vi "Read.vi"(8 "error in":errorcluster, 11 "VISA resource name":refnum<visa-resource-name>) -> (0 "error out":errorcluster, 2 "Message":string, 3 "VISA resource name out":refnum<visa-resource-name>)   [LabVIEW 2019, in "Andeen-Hagerling 2700(400 firmware).lvlib"]
doc: "Read all available bytes from the selected VISA resource."
uses:
  Andeen-Hagerling 2700(400 firmware).lvlib
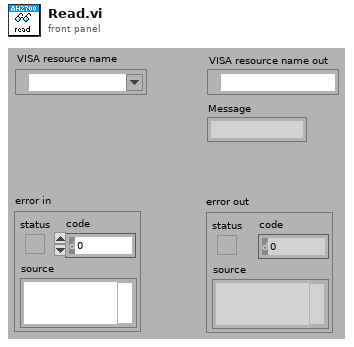
[diagram p1: front panel]
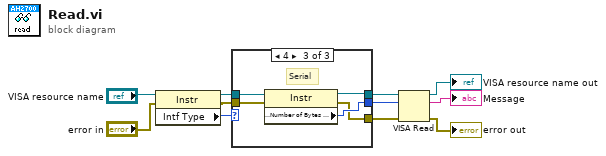
[diagram p0: block diagram]
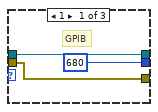
[diagram p2: hidden frame]
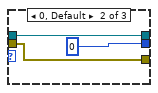
[diagram p3: hidden frame]
diagram:
  n1 = property class="Instr"(reference="VISA resource name", error in="error in") -> (reference out=w10:refnum<visa-resource-name>, error out=w4:errorcluster, "Intf Type"=w11:u16)
  n2 = case shown="4" w11 {
    tunnel: w10 -> [w13 w17 w22]
    tunnel: [w13 w17 w20] -> w9
    tunnel: [w12 w15 w19] -> w8
    tunnel: [u16 680 ("y") u32 0 ("Bytes at Port") w21] -> w7
    tunnel: w4 -> [w12 w15 w18]
    frame 1 {
      # "GPIB"
    }
    frame 0, Default {
    }
    frame 4 {
      # "Serial"
      n3 = property class="Instr"(reference=w22, error in=w18) -> (reference out=w20:refnum<visa-resource-name>, error out=w19:errorcluster, "Serial Settings:Number of Bytes at Serial Port"=w21:u32)
    }
  }
  n4 = VISA Read(VISA resource name=w9, byte count=w7, error in (no error)=w8) -> (VISA resource name out=→"VISA resource name out":refnum<visa-resource-name>, read buffer=→"Message":string, error out=→"error out":errorcluster)  [unwired: 1 out]
